vi "MathCad_File_Open.vi"(8 "error in (no error)":errorcluster, 10 "Worksheet File":path, 11 "Mathcad.IMathcadApplication":refnum<k7>) -> (0 "error out (no error)":errorcluster, 1 "Worksheet Reference":refnum<k7>, 2 "Worksheets Reference":refnum<k7>, 3 "Application Reference":refnum<k7>)   [LabVIEW 2015]
doc: "Opens a Mathcad File (*.mcd).\n\nInputs\nMathcad Application Reference- Reference to the Mathcad Application Classs\nFile Name (String)-File path to *.mcd file to open\n\nOutputs\n\nMathcad Application Reference- Reference to the Mathcad Application Class\nWorksheets Reference-Reference to the Worksheets Class that contains the Worksheet (*.mcd file) that was opened\nWorksheet Reference-Reference to the Worksheet Class that was opened to the file."
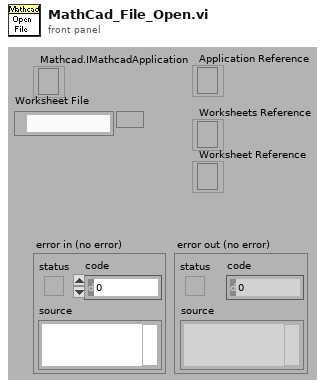
[diagram p1: front panel]
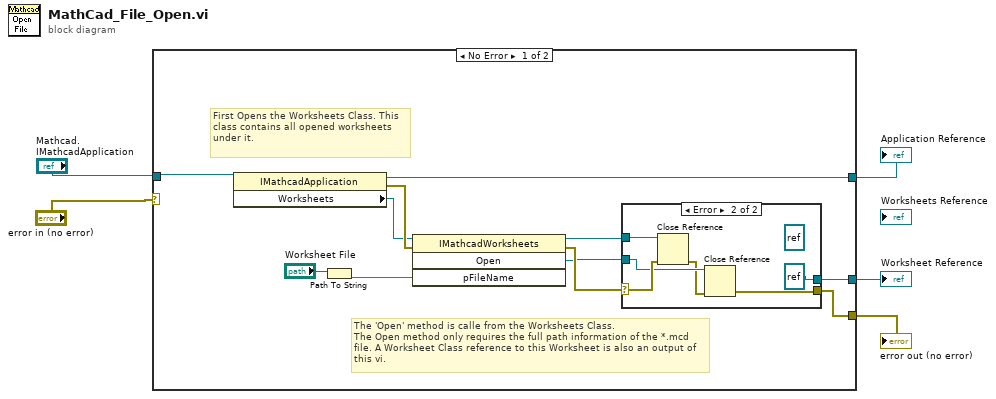
[diagram p0: block diagram]
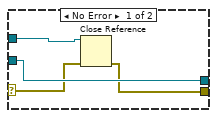
[diagram p2: hidden frame]
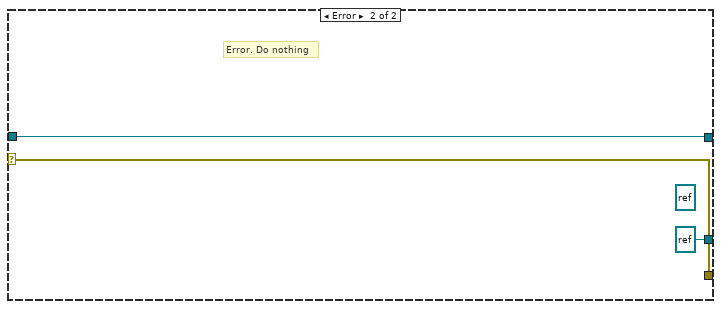
[diagram p3: hidden frame]
diagram:
  n1 = case shown="No Error" "error in (no error)" {
    selector: "error in (no error)" -> [_ w29]
    tunnel: [w9 w29] -> w5
    tunnel: [w15 w28] -> w3
    tunnel: "Mathcad.IMathcadApplication" -> [w14 w28]
    tunnel: [w8 refnum<k7> refnum ("Open")] -> w1
    frame No Error {
      # "The 'Open' method is calle from the Worksheets Class.\nThe Open method only requires the full path information of the *.mcd file. A Worksheet Class reference to this Worksheet is also an output of this vi."
      # "First Opens the Worksheets Class. This class contains all opened worksheets under it."
      n2 = property class="IMathcadApplication"(reference=w14) -> (reference out=w15:refnum<k7>, error out=w16:errorcluster, "Worksheets"=w13:refnum<k7>)  [unwired: 1 in]
      n3 = Path To String(path="Worksheet File") -> (string=w6:string)
      n4 = invoke class="IMathcadWorksheets" method="Open"(reference=w13, error in=w16, "pFileName"=w6) -> (reference out=w11:refnum<k7>, error out=w12:errorcluster, "Open"=w10:refnum<k7>)  [unwired: 1 in, 1 out]
      n5 = case shown="Error" w12 {
        selector: w12 -> [w18 w25]
        tunnel: w11 -> [w19 w26]
        tunnel: w10 -> [w20 w24]
        tunnel: [w17 w22] -> w9
        tunnel: [w20 refnum<k7> refnum ("Open")] -> w8
        frame No Error {
          n6 = Close Reference(reference=w19, error in (no error)=w18) -> (error out=w17:errorcluster)
        }
        frame Error {
          (unwired) refnum<k7> refnum ("Worksheets")
          n7 = Close Reference(reference=w26, error in (no error)=w25) -> (error out=w23:errorcluster)
          n8 = Close Reference(reference=w24, error in (no error)=w23) -> (error out=w22:errorcluster)
        }
      }
    }
    frame Error {
      (unwired) refnum<k7> refnum ("Worksheets")
      # "Error. Do nothing"
    }
  }
  "error out (no error)" <- w5
  "Application Reference" <- w3
  "Worksheet Reference" <- w1
